vi "数据查询.vi"() -> ()   [LabVIEW 2016, in "数据查询.lvlib"]
uses:
  <vilib>/Utility/miscctls.llb/LVPointTypeDef.ctl
panel:
  in  "标识说明":bool
  in  "数据查询菜单":enum32{"数据查询", "仪器数据", "仪器日志", "报警信息", "校准日志"}(xcontrol)
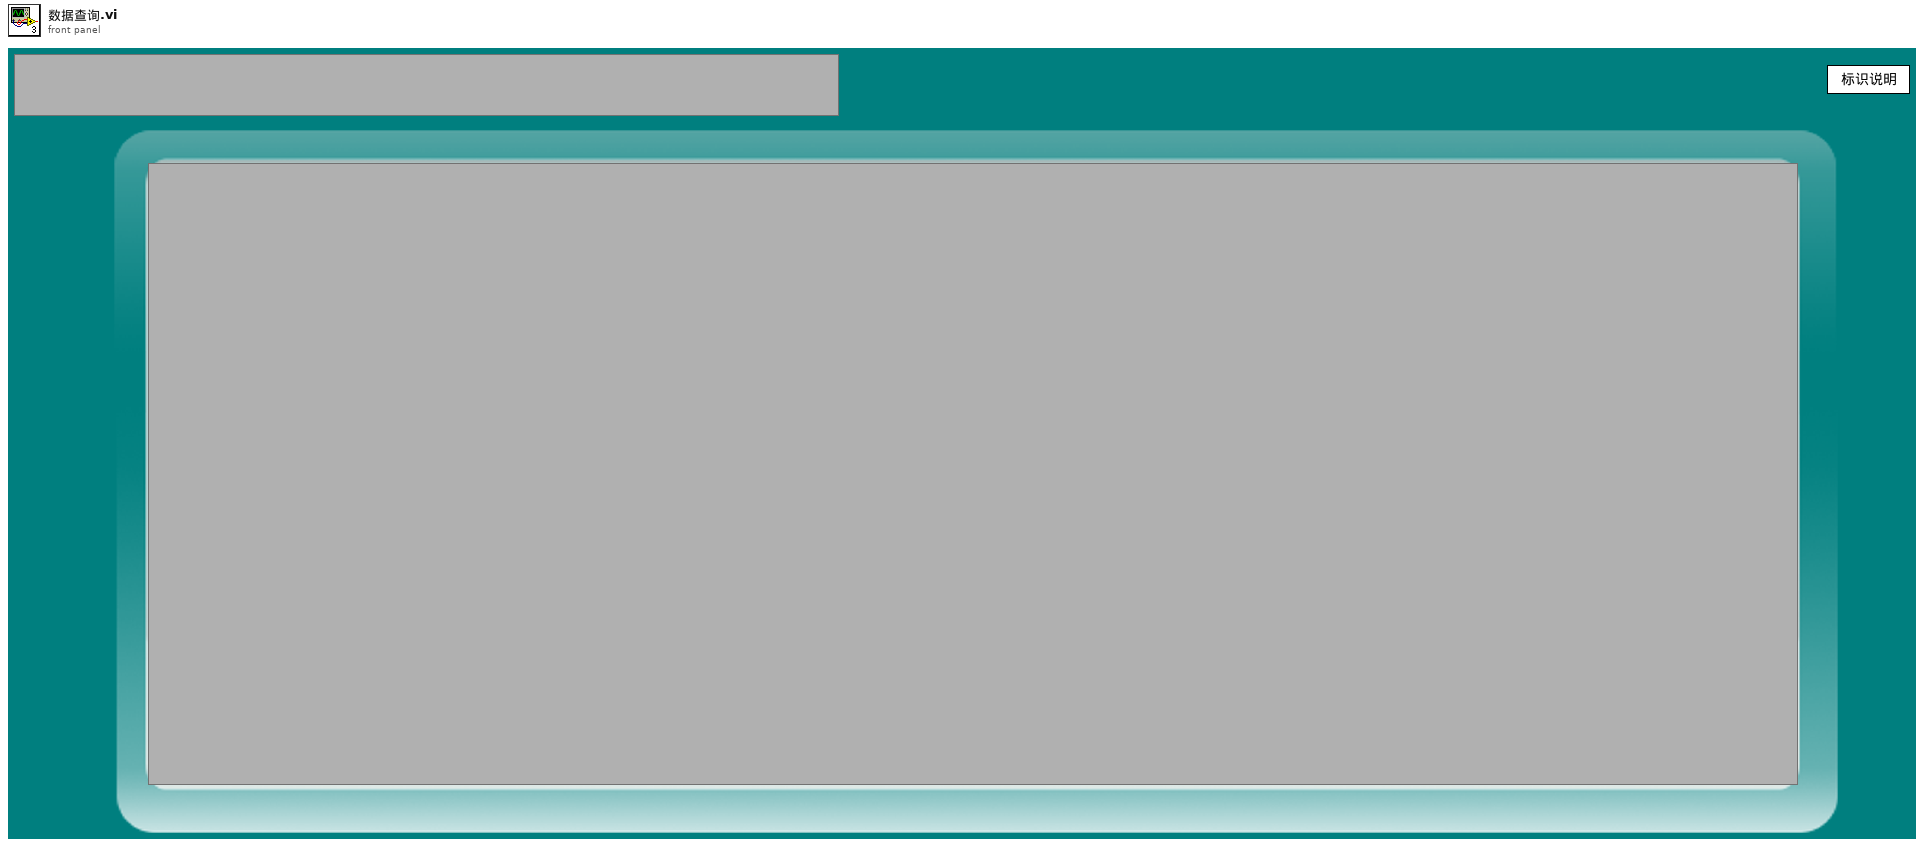
[diagram p1: front panel]
types:
  T1 = typedef "LVPointTypeDef.ctl" = cluster{"Horizontal":i16, "Vertical":i16}
  T2 = typedef "LVDateTimeRec.ctl" = cluster{"秒数的小数部分":dbl, "秒":i32, "分":i32, "时":i32, "日":i32, "月":i32, "年":i32, "天数（周）":i32, "天数（年）":i32, "DST":i32}
  T3 = enum32{"Bad", "Idle", "Run top level", "Running"}
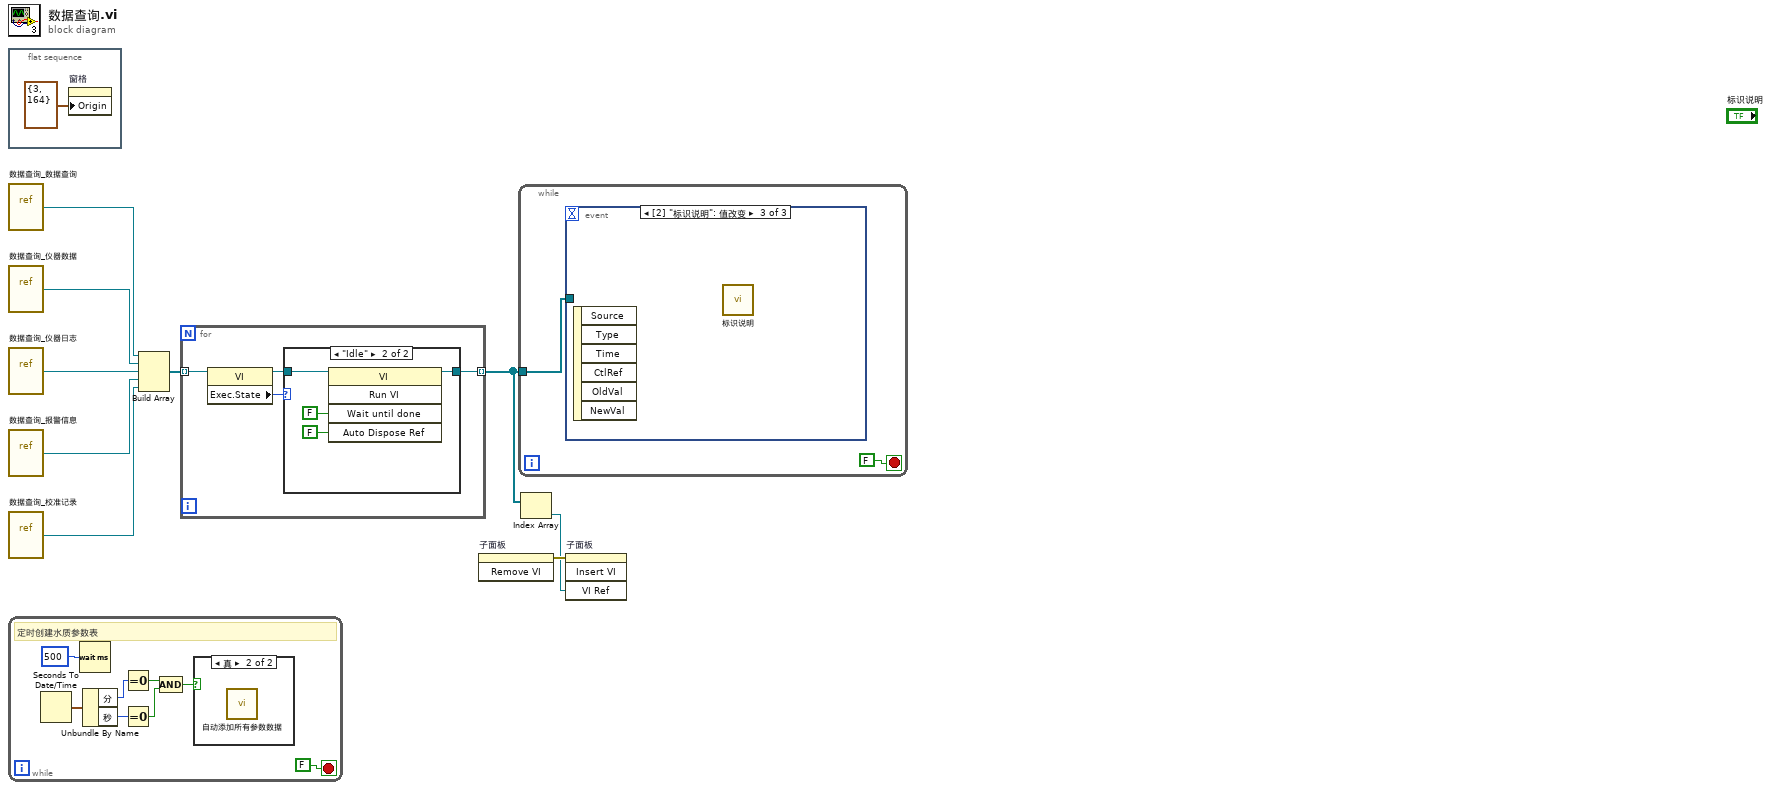
[diagram p0: block diagram]
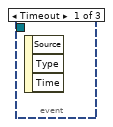
[diagram p4: hidden frame]
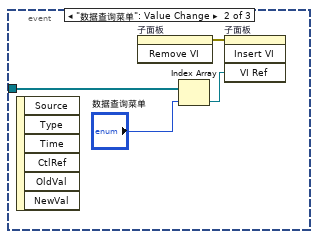
[diagram p5: hidden frame]
diagram:
  n1 = flat-sequence {
    frame #0 {
      n2 = property on="窗格" class="Pane"("Origin"=T1 {"Horizontal"=3, "Vertical"=164} ("原点")) -> ()  [unwired: 2 in, 2 out]
    }
  }
  n3 = vi-ref "数据查询_数据查询.vi"() -> (w6:refnum<vi>)
  n4 = vi-ref "数据查询_仪器数据.vi"() -> (w4:refnum<vi>)
  n5 = vi-ref "数据查询_仪器日志.vi"() -> (w3:refnum<vi>)
  n6 = vi-ref "数据查询_报警信息.vi"() -> (w2:refnum<vi>)
  n7 = vi-ref "数据查询_校准记录.vi"() -> (w1:refnum<vi>)
  n8 = while {
    stop <- FALSE stop-if-true
    # "定时创建水质参数表"
    n9 = Seconds To Date/Time() -> (date time rec=w18:T2)  [unwired: 2 in]
    n10 = Wait (ms)(milliseconds to wait=u32 500 ("等待时间（毫秒）")) -> ()  [unwired: 1 out]
    n11 = Unbundle By Name(w18) -> ("分"=w17:i32, "秒"=w16:i32)
    n12 = Equal To 0?(x=w17) -> (x = 0?=w15:bool)
    n13 = Equal To 0?(x=w16) -> (x = 0?=w14:bool)
    n14 = Compound Arithmetic op=AND ("复合运算")(w15, w14) -> (w13:bool)
    n15 = case shown="真" w13 {
      frame False {
      }
      frame True {
        n16 = call "自动添加所有参数数据.vi"() -> ()  [unwired: 12 in]
      }
    }
  }
  n17 = Build Array(w6, w4, w3, w2, w1) -> (w5:refnum<vi>[])
  n18 = for {
    tunnel: w5 -> [w22] mode=indexing
    tunnel: [w19] -> w8 mode=indexing
    n19 = property class="VI"(reference=w22) -> (reference out=w20:refnum<vi>, "Exec.State"=w21:T3)  [unwired: 1 in, 1 out]
    n20 = case shown="\"Idle\"" w21 {
      tunnel: w20 -> [w23 w25]
      tunnel: [w23 w24] -> w19
      frame "Bad", Default {
      }
      frame "Idle" {
        n21 = invoke class="VI" method="Run VI"(reference=w25, "Wait until done"=FALSE ("结束前等待"), "Auto Dispose Ref"=FALSE ("自动销毁引用")) -> (reference out=w24:refnum<vi>)  [unwired: 2 in, 4 out]
      }
    }
  }
  n22 = invoke on="子面板" class="SubPnl" method="Remove VI"() -> (error out=w9:errorcluster)  [unwired: 3 in, 2 out]
  n23 = while {
    tunnel: w8 -> [w28]
    stop <- FALSE stop-if-true
    n24 = event shown="[2] \"标识说明\": 值改变" {
      selector: _ -> [_ _ _]
      dyn-events: _ -> [_ _ _]
      timeout: _ -> [_ _ _]
      tunnel: w28 -> [_ w33 _]
      event Timeout {
        n25 = event-data() -> ()  [unwired: 1 in, 3 out]
      }
      event "数据查询菜单": Value Change {
        n26 = event-data() -> ()  [unwired: 1 in, 6 out]
        n27 = invoke on="子面板" class="SubPnl" method="Remove VI"() -> (error out=w30:errorcluster)  [unwired: 3 in, 2 out]
        n28 = Index Array(array=w33, index="数据查询菜单") -> (element=w31:refnum<vi>)
        n29 = invoke on="子面板" class="SubPnl" method="Insert VI"(error in=w30, "VI Ref"=w31) -> ()  [unwired: 2 in, 4 out]
      }
      event "标识说明": Value Change {
        n30 = event-data() -> ()  [unwired: 1 in, 6 out]
        n31 = call "标识说明.vi"() -> ()  [unwired: 12 in]
      }
    }
  }
  n32 = Index Array(array=w8) -> (element=w7:refnum<vi>)  [unwired: 1 in]
  n33 = invoke on="子面板" class="SubPnl" method="Insert VI"(error in=w9, "VI Ref"=w7) -> ()  [unwired: 2 in, 4 out]
